vi "斯坦道XML解析.vi"(10 "添加的路径":path, 11 "参数簇":cluster{"启动模式":u16, "启动参数":u16, "量程":u16}={"启动模式"=0, "启动参数"=1, "量程"=0} {"量程" items=["低量程", "高量程"]; "启动参数" items=["CODMn"=21, "总氮"=2, "氨氮"=3]; "启动模式" items=["", "水样测量", "标样核查", "零点核查", "跨度核查", "空白测试", "平行样测试", "加标回收", "校零", "校标"]}) -> (2 "步骤时间":string[](array[string]), 3 "步骤名":string[](array[string]))   [LabVIEW 2016, in "斯坦道CODMn新电路板.lvlib"]
uses:
  <vilib>/xml/Load XML File.vi
  <vilib>/xml/Close Reference(Node).vi
  <resource>/objmgr/DOMUserDefRef.rc
  <vilib>/xml/NI_XML.lvlib
panel:
  out "连接的字符串":string
  out "大小":i32
  out "XML字符串":string="<?xml version=\"1.0\" encoding=\"ISO-8859-1\"?>\n<bookstore>\n<book ISBN=\"978-0545128285\">\n  <title lang=\"en\">The Tales of Beedle the Bard</title>\n  <author>J. K. Rowling</author>\n  <year>2008</year>\n  <price>12.99</price>\n</book>\n<book ISBN=\"978-0316160209\">\n  <title lang=\"en\">Eclipse</title>\n  <author>Stephenie Meyer</author>\n  <year>2007</year>\n  <price>19.99</price>\n</book>\n<book ISBN=\"978-0316067928\">\n  <title lang=\"en\">Breaking Dawn</title>\n  <author>Stephenie Meyer</author>\n  <year>2008</year>\n  <price>22.99</price>\n</book>\n<book ISBN=\"978-0316017923\">\n  <title lang=\"en\">Outliers: The Story of Success</title>\n  <author>Malcolm Gladwell</author>\n  <year>2008</year>\n  <price>27.99</price>\n</book>\n<book ISBN=\"978-0596007645\">\n  <title lang=\"en\">XML in a Nutshell</title>\n  <author>Elliotte Rusty Harold</author>\n  <author>W. Scott Means</author>\n  <year>2004</year>\n  <price>39.95</price>\n</book>\n</bookstore>"
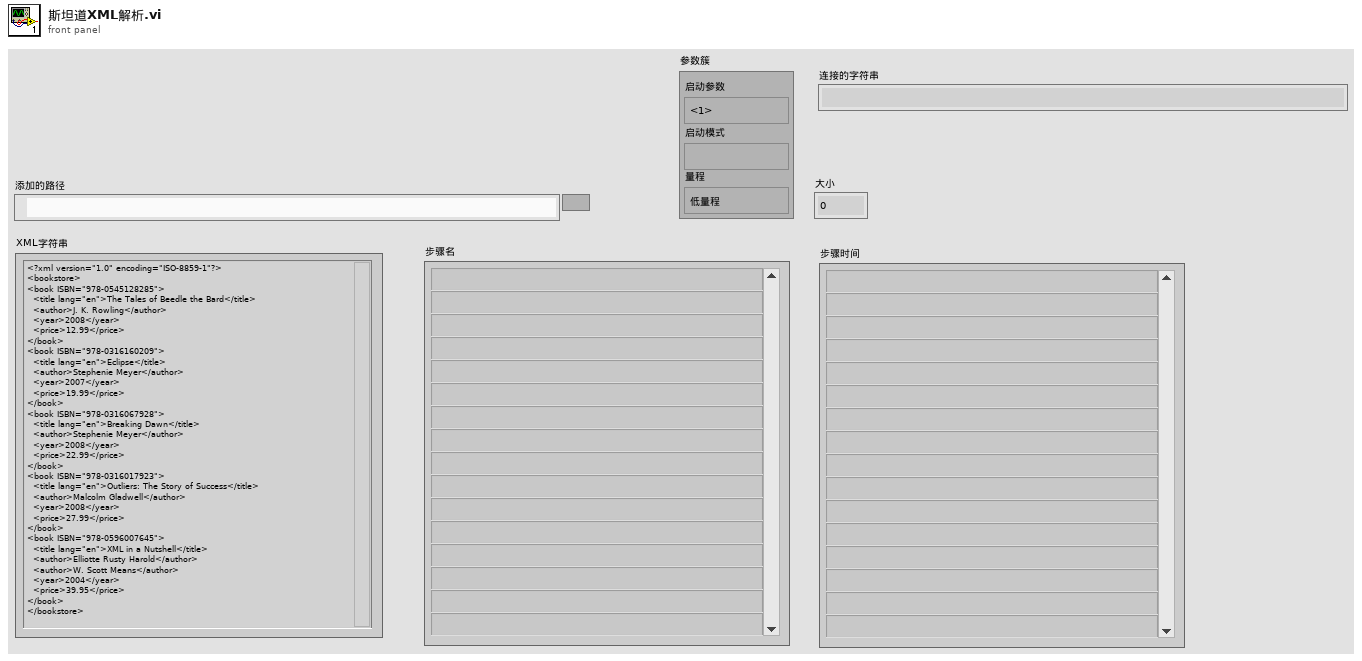
[diagram p1: front panel]
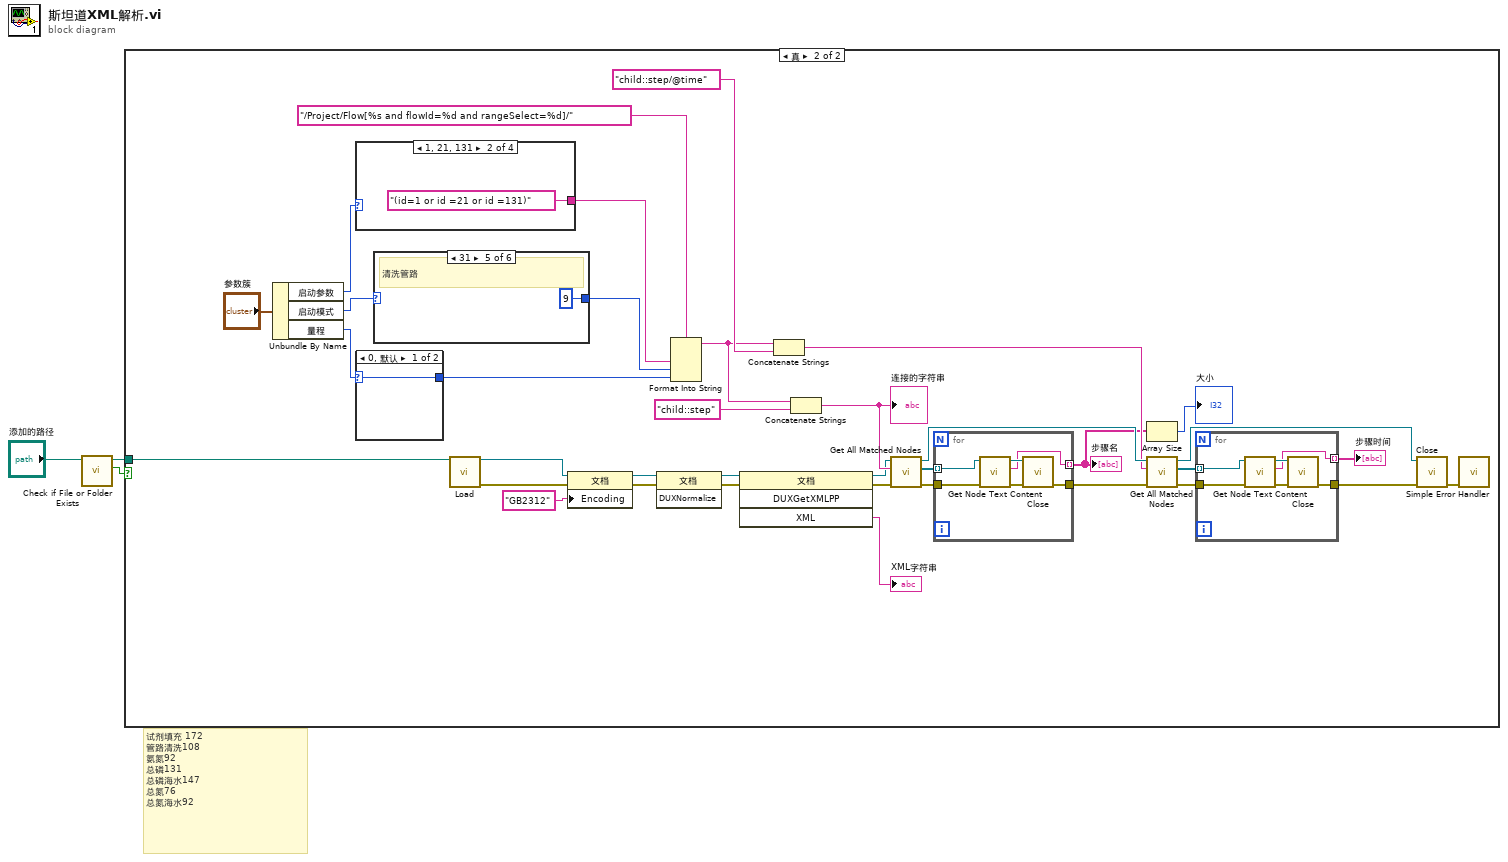
[diagram p0: block diagram]
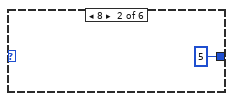
[diagram p4: hidden frame]
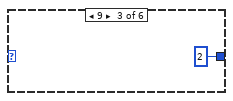
[diagram p5: hidden frame]
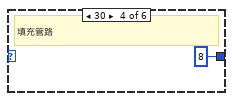
[diagram p6: hidden frame]
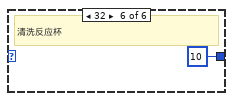
[diagram p7: hidden frame]
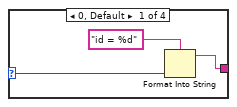
[diagram p8: hidden frame]
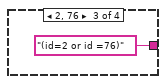
[diagram p9: hidden frame]
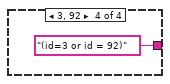
[diagram p10: hidden frame]
diagram:
  # "试剂填充 172 \n管路清洗108\n氨氮92\n总磷131\n总磷海水147\n总氮76\n总氮海水92"
  n1 = call <vilib>:"Check if File or Folder Exists.vi"("path"="添加的路径") -> ("file or folder exists?"=w1:bool, "dup path"=w2:path)  [unwired: 8 in, 1 out]
  n2 = case shown="真" w1 {
    tunnel: w2 -> [_ w6]
    frame False {
    }
    frame True {
      n3 = Unbundle By Name("参数簇") -> ("启动参数"=w8:u16, "启动模式"=w5:u16, "量程"=w11:u16)
      n4 = case shown="1, 21, 131" w8 {
        selector: w8 -> [w47 _ _ _]
        tunnel: [w46 "(id=1 or id =21 or id =131)" ("输入 4") "(id=2 or id =76)" ("输入 4") "(id=3 or id = 92)" ("输入 4")] -> w7
        frame 0, Default {
          n5 = Format Into String(format string="id = %d" ("格式字符串"), w47) -> (resulting string=w46:string)  [unwired: 2 in, 1 out]
        }
        frame 1, 21, 131 {
        }
        frame 2, 76 {
        }
        frame 3, 92 {
        }
      }
      n6 = case shown="0, 默认" w11 {
        selector: w11 -> [w58 w59]
        tunnel: [w58 w59] -> w28
        frame 0, Default {
        }
        frame 1 {
        }
      }
      n7 = case shown="31" w5 {
        selector: w5 -> [w40 _ _ _ _ _]
        tunnel: [w40 u16 5 ("启动模式") u16 2 ("启动模式") u16 8 ("启动模式") u16 9 ("启动模式") u16 10 ("启动模式")] -> w4
        frame 0, Default {
        }
        frame 8 {
        }
        frame 9 {
        }
        frame 30 {
          # "填充管路"
        }
        frame 31 {
          # "清洗管路"
        }
        frame 32 {
          # "清洗反应杯"
        }
      }
      n8 = call-poly <vilib>:"Load.vi"("path to XML document"=w6) -> ("DOM document out"=w37:refnum<k20>, "error out"=w36:errorcluster)  [unwired: 12 in, 1 out]
      n9 = property on="属性节点" class="文档"(reference=w37, error in=w36, "Encoding"="GB2312" ("文档编码")) -> (reference out=w35:refnum<k20>, error out=w34:errorcluster)
      n10 = invoke on="Invoke Node" class="文档" method="DUXNormalize"(reference=w35, error in=w34) -> (reference out=w32:refnum<k20>, error out=w33:errorcluster)  [unwired: 1 in, 1 out]
      n11 = Format Into String(format string="/Project/Flow[%s and flowId=%d and rangeSelect=%d]/" ("XPath expression"), w7, w4, w28) -> (resulting string=w17:string)  [unwired: 2 in, 1 out]
      n12 = invoke on="Invoke Node" class="文档" method="DUXGetXMLPP"(reference=w32, error in=w33) -> (reference out=w14:refnum<k20>, error out=w15:errorcluster, "XML"=→"XML字符串":string)  [unwired: 2 in, 1 out]
      n13 = Concatenate Strings(w17, "child::step/@time" ("输入 4")) -> (w18:string)
      n14 = Concatenate Strings(w17, "child::step" ("输入 4")) -> (w20:string)
      "连接的字符串" <- w20
      n15 = call <vilib>:"Get All Matched Nodes.vi"("error in (no error)"=w15, "XPath expression"=w20, "node in"=w14) -> ("error out"=w31:errorcluster, "node result array"=w30:refnum<k20>[], "node out"=w24:refnum<k20>)  [unwired: 6 in]
      n16 = for {
        tunnel: w31 -> [w65]
        tunnel: [w62] -> w10 mode=indexing
        tunnel: w30 -> [w61] mode=indexing
        tunnel: [w60] -> w23
        n17 = call <vilib>:"Get Node Text Content.vi"("error in (no error)"=w65, "node in"=w61) -> ("error out"=w63:errorcluster, "node text"=w62:string, "node out"=w64:refnum<k20>)  [unwired: 7 in]
        n18 = call-poly <vilib>:"Close.vi"("error in (no error)"=w63, "node"=w64) -> ("error out"=w60:errorcluster)  [unwired: 7 out]
      }
      "步骤名" <- w10
      n19 = Array Size(array=w10) -> (size(s)=→"大小":i32)
      n20 = call <vilib>:"Get All Matched Nodes.vi"("error in (no error)"=w23, "XPath expression"=w18, "node in"=w24) -> ("error out"=w26:errorcluster, "node result array"=w25:refnum<k20>[], "node out"=w13:refnum<k20>)  [unwired: 6 in]
      n21 = for {
        tunnel: w26 -> [w57]
        tunnel: [w54] -> w22 mode=indexing
        tunnel: w25 -> [w53] mode=indexing
        tunnel: [w52] -> w16
        n22 = call <vilib>:"Get Node Text Content.vi"("error in (no error)"=w57, "node in"=w53) -> ("error out"=w55:errorcluster, "node text"=w54:string, "node out"=w56:refnum<k20>)  [unwired: 7 in]
        n23 = call-poly <vilib>:"Close.vi"("error in (no error)"=w55, "node"=w56) -> ("error out"=w52:errorcluster)  [unwired: 7 out]
      }
      "步骤时间" <- w22
      n24 = call-poly <vilib>:"Close.vi"("error in (no error)"=w16, "node"=w13) -> ("error out"=w27:errorcluster)  [unwired: 7 out]
      n25 = call <vilib>:"Simple Error Handler.vi"("error in (no error)"=w27) -> ()  [unwired: 4 in, 5 out]
    }
  }
